vi "Gamma CDF.vi"(9 "c":dbl=1.0, 10 "b":dbl=1.0, 11 "x":dbl=1.0) -> (0 "error":i32, 3 "cdf(x)":dbl=0.6321205588285578)   [LabVIEW 2018, in "NI_Gmath.lvlib"]
doc: "Computes the continuous cumulative distribution function (CDF), or the probability that the random variate X, where X describes the selected distribution type, has a value less than or equal to <B>x</B>. You must manually select the polymorphic instance to use."
uses:
  NI_Gmath.lvlib
  st_error_code.ctl
  Incomplete Gamma Function.vi
panel:
  # "Gamma CDF"
  # "scale"
  # "shape"
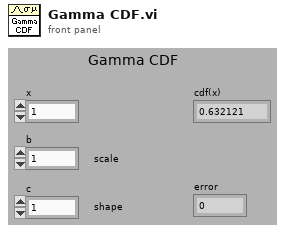
[diagram p1: front panel]
types:
  T1 = typedef "NI_Gmath.lvlib/st_error_code.ctl" = i32
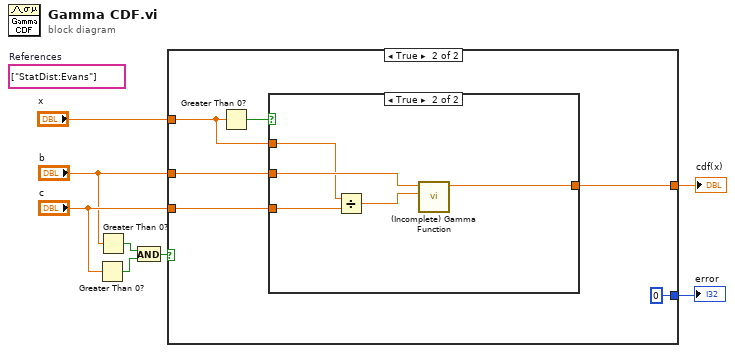
[diagram p0: block diagram]
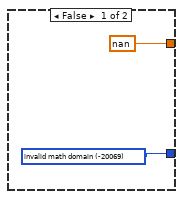
[diagram p2: hidden frame]
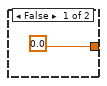
[diagram p3: hidden frame]
diagram:
  (unwired) string[] ["StatDist:Evans"]  # References
  n1 = Greater Than 0?(x="c") -> (x > 0?=w2:bool)
  n2 = Greater Than 0?(x="b") -> (x > 0?=w1:bool)
  n3 = And(x=w1, y=w2) -> (x .and. y?=w5:bool)
  n4 = case shown="True" w5 {
    tunnel: "c" -> [_ w11]
    tunnel: [w9 0 ("invalid math domain")] -> w8
    tunnel: [nan w14] -> w7
    tunnel: "x" -> [_ w13]
    tunnel: "b" -> [_ w12]
    frame False {
      w9 = T1 -20069 items=["invalid math domain"=-20069, "Fourier interpolation size m >= n"=-20070, "empty array"=-20003] ("stat interp error code")
    }
    frame True {
      n5 = Greater Than 0?(x=w13) -> (x > 0?=w15:bool)
      n6 = case shown="True" w15 {
        tunnel: [0.0 w19] -> w14
        tunnel: w13 -> [_ w21]
        tunnel: w12 -> [_ w22]
        tunnel: w11 -> [_ w20]
        frame False {
        }
        frame True {
          n7 = Divide(x=w21, y=w20) -> (x/y=w18:dbl)
          n8 = call-poly "(Incomplete) Gamma Function.vi"("a"=w18, "x"=w22) -> ("g(x, a)"=w19:dbl)  [unwired: 9 in]
        }
      }
    }
  }
  "cdf(x)" <- w7
  "error" <- w8
